vi "InitMultipleDevices.vi"(4 "error in (no error)":errorcluster, 6 "msecDelayForDiscovery":i32, 7 "logging":bool) -> (0 "error out":errorcluster, 2 "DeviceKey List Out":string[](array[string]), 3 "CmdLib Out":refnum<k24>)   [LabVIEW 2012]
uses:
  D:/workspace/GitHub/LVsolis/lib/CmdLib.dll
  lib/CmdLib.dll
panel:
  in  "deviceKey":string
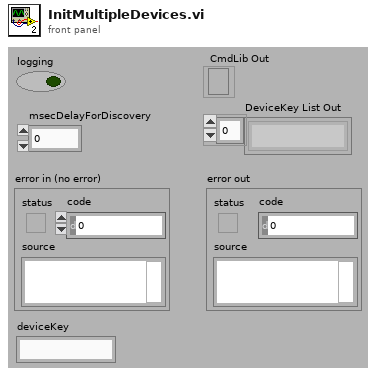
[diagram p1: front panel]
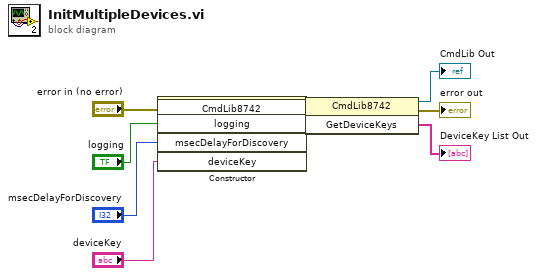
[diagram p0: block diagram]
diagram:
  n1 = constructor class="CmdLib8742"(error in="error in (no error)", "logging"="logging", "msecDelayForDiscovery"="msecDelayForDiscovery", "deviceKey"="deviceKey") -> (reference out=w5:refnum<k24>, error out=w4:errorcluster)  [unwired: 2 in, 4 out]
  n2 = invoke class="CmdLib8742" method="GetDeviceKeys"(reference=w5, error in=w4) -> (reference out=→"CmdLib Out":refnum<k24>, error out=→"error out":errorcluster, "GetDeviceKeys"=→"DeviceKey List Out":string[])  [unwired: 1 in]
